vi "Create Instrument Addon From Configuration File.vi"(8 "error in (no error)":errorcluster, 10 "configuration file path":path, 11 "target in":refnum<k24>) -> (0 "error out":errorcluster, 2 "instrument addon refnum":T1=18446744073709551615 format="%.0x", 3 "target out":refnum<k24>)   [LabVIEW 2019, in "Scripting API.lvlib"]
uses:
  Scripting API.lvlib
  NationalInstruments.VeriStand.SystemDefinitionAPI
  <vilib>/NI VeriStand/Custom Device API/Custom Device Item Ref.ctl
  <vilib>/NI VeriStand/Custom Device API/Custom Device API.lvlib
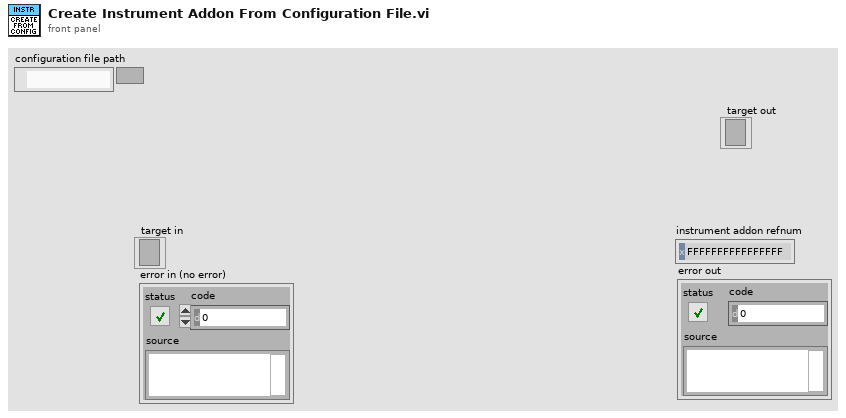
[diagram p1: front panel]
types:
  T1 = typedef "Custom Device API.lvlib/Custom Device Item Ref.ctl" = u64
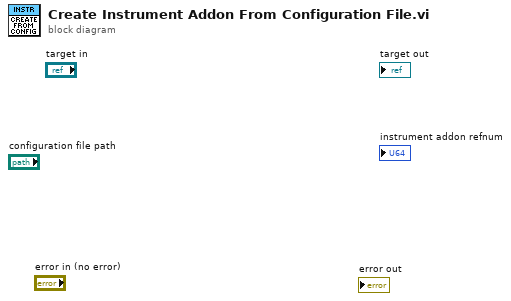
[diagram p0: block diagram]
diagram:
